vi "RailPress_PID.vi"(0 "Control Enable":bool, 1 "Fault Input":bool, 2 "Rail Press Setpoint":sgl format="%.2f", 3 "Rail Pressure":sgl format="%.2f", 5 "PID Enable":bool, 9 "PID Settings":T5={"PID_Kp"=0.0, "PID_Ti"=0.01, "PID_Td"=0.0, "PID_FF"=0.0, "Non-PID_FF"=0.0, "PID_Min"=-100.0, "PID_Max"=100.0} {"PID_Max" format="%.2f"; "PID_Min" format="%.2f"; "PID_Td" format="%.3f"; "PID_Ti" format="%.3f"}, 11 "Output Management Controls":T3, 12 "dt (s)":sgl=-1.0 format="%.3f") -> (4 "Output":T4, 14 "PID_Action_Output":T2, 15 "LS Output":T1)   [LabVIEW 2015, in "ECS-RT.lvlib"]
uses:
  ECS-RT.lvlib
  Typedefs/Raw Outputs/LS.ctl
  ECS-Shared.lvlib
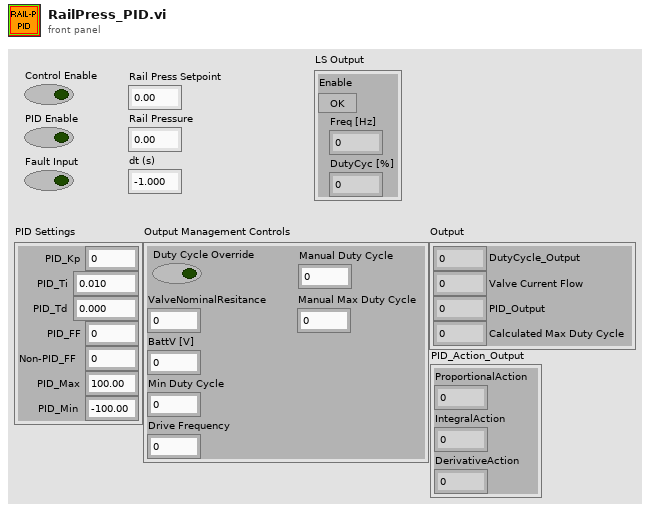
[diagram p1: front panel]
types:
  T1 = typedef "ECS-Shared.lvlib/LS.ctl" = cluster{"Enable":bool, "Freq [Hz]":sgl, "DutyCyc [%]":sgl}
  T2 = cluster{"ProportionalAction":sgl, "IntegralAction":sgl, "DerivativeAction":sgl}
  T3 = cluster{"BattV [V]":sgl, "ValveNominalResitance":sgl, "Min Duty Cycle":sgl, "Manual Max Duty Cycle":sgl, "Manual Duty Cycle":sgl, "Duty Cycle Override":bool, "Drive Frequency":sgl}
  T4 = cluster{"DutyCycle_Output":sgl, "Calculated Max Duty Cycle":sgl, "Valve Current Flow":sgl, "PID_Output":sgl}
  T5 = cluster{"PID_Kp":sgl, "PID_Ti":sgl, "PID_Td":sgl, "PID_FF":sgl, "Non-PID_FF":sgl, "PID_Min":sgl, "PID_Max":sgl}
  T6 = cluster{"DutyCycle_Output":sgl, "Max Duty Cycle":sgl, "Valve Current Flow":sgl, "PID_Output":sgl}
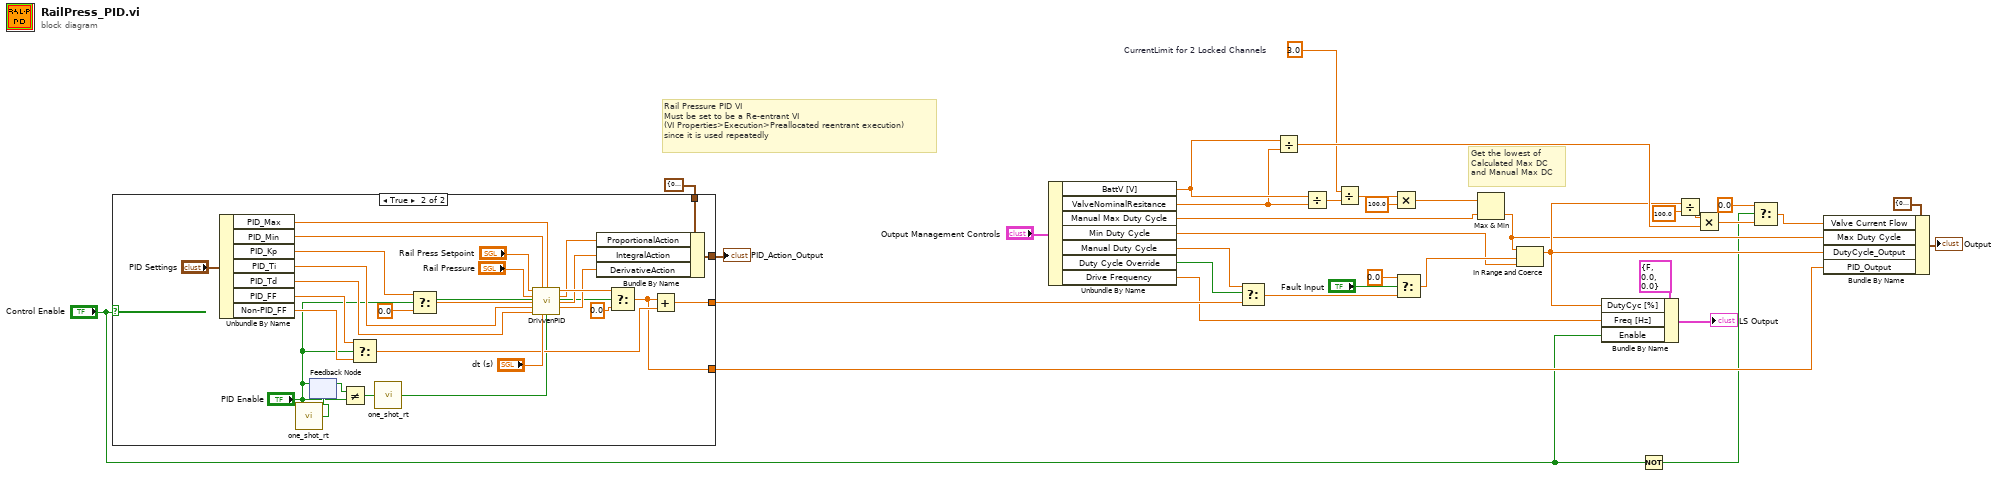
[diagram p0: block diagram]
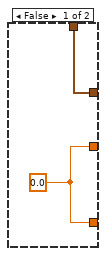
[diagram p2: hidden frame]
diagram:
  w4 = sgl 3.0  # CurrentLimit for 2 Locked Channels
  # "Rail Pressure PID VI\nMust be set to be a Re-entrant VI \n(VI Properties>Execution>Preallocated reentrant execution)\nsince it is used repeatedly"
  # "Get the lowest of \nCalculated Max DC\nand Manual Max DC"
  n1 = case shown="True" "Control Enable" {
    tunnel: [w37 w57] -> w19
    tunnel: [w37 w54] -> w23
    tunnel: T2 {"ProportionalAction"=0.0, "IntegralAction"=0.0, "DerivativeAction"=0.0} -> [w36 w43]
    tunnel: [w36 w42] -> w11
    frame False {
      w37 = sgl 0.0 ("f")
    }
    frame True {
      n2 = Unbundle By Name("PID Settings") -> ("PID_Max"=w50:sgl, "PID_Min"=w49:sgl, "PID_Kp"=w51:sgl, "PID_Ti"=w48:sgl, "PID_Td"=w47:sgl, "PID_FF"=w46:sgl, "Non-PID_FF"=w45:sgl)
      n3 = call <vilib>:"one_shot_rt.vi"("I"="PID Enable") -> ("O"=w39:bool)
      n4 = feedback #1(w39) -> (w56:bool)
      n5 = feedback-in #1("PID Enable") -> ()
      n6 = Not Equal?(x=w56, y="PID Enable") -> (x != y?=w55:bool)
      n7 = Select(t=w46, s="PID Enable", f=w45) -> (s? t:f=w60:sgl)
      n8 = call <vilib>:"one_shot_rt.vi"("I"=w55) -> ("O"=w53:bool)
      n9 = Select(t=w51, s="PID Enable", f=sgl 0.0 ("t")) -> (s? t:f=w64:sgl)
      n10 = call <vilib>:"DrivvenPID.vi"("Setpoint"="Rail Press Setpoint", "OutputLow"=w49, "OutputHigh"=w50, "ProcessVariable"="Rail Pressure", "ProportionalGain (Kc)"=w64, "IntegralTime (Ti, min)"=w48, "DerivativeTime (Td, min)"=w47, "dt (s)"="dt (s)", "Reinitialize? (F)"=w53) -> ("Output"=w59:sgl, "ProportionalAction"=w44:sgl, "IntegralAction"=w41:sgl, "DerivativeAction"=w40:sgl)  [unwired: 1 in, 2 out]
      n11 = Bundle By Name(cluster=w43, "ProportionalAction"=w44, "IntegralAction"=w41, "DerivativeAction"=w40) -> (w42:T2)
      n12 = Select(t=w59, s="PID Enable", f=sgl 0.0) -> (s? t:f=w57:sgl)
      n13 = Add(x=w57, y=w60) -> (x+y=w54:sgl)
    }
  }
  "PID_Action_Output" <- w11
  n14 = Unbundle By Name("Output Management Controls") -> ("BattV [V]"=w9:sgl, "ValveNominalResitance"=w8:sgl, "Manual Max Duty Cycle"=w6:sgl, "Min Duty Cycle"=w17:sgl, "Manual Duty Cycle"=w16:sgl, "Duty Cycle Override"=w15:bool, "Drive Frequency"=w13:sgl)
  n15 = Select(t=w16, s=w15, f=w23) -> (s? t:f=w25:sgl)
  n16 = Divide(x=w9, y=w8) -> (x/y=w32:sgl)
  n17 = Divide(x=w9, y=w8) -> (x/y=w31:sgl)
  n18 = Divide(x=w4, y=w31) -> (x/y=w30:sgl)
  n19 = Multiply(x=w30, y=sgl 100.0) -> (x*y=w7:sgl)
  n20 = Select(t=sgl 0.0, s="Fault Input", f=w25) -> (s? t:f=w24:sgl)
  n21 = Max & Min(x=w7, y=w6) -> (min(x,y)=w5:sgl)  [unwired: 1 out]
  n22 = In Range and Coerce(upper limit=w5, x=w24, lower limit=w17) -> (coerced(x)=w14:sgl)  [unwired: 1 out]
  n23 = Bundle By Name(cluster=T1 {"Enable"=FALSE, "Freq [Hz]"=0.0, "DutyCyc [%]"=0.0} ("LS Output"), "DutyCyc [%]"=w14, "Freq [Hz]"=w13, "Enable"="Control Enable") -> (→"LS Output":T1)
  n24 = Not(x="Control Enable") -> (.not. x?=w1:bool)
  n25 = Divide(x=w14, y=sgl 100.0) -> (x/y=w33:sgl)
  n26 = Multiply(x=w33, y=w32) -> (x*y=w35:sgl)
  n27 = Select(t=sgl 0.0, s=w1, f=w35) -> (s? t:f=w20:sgl)
  n28 = Bundle By Name(cluster=T6 {"DutyCycle_Output"=0.0, "Max Duty Cycle"=0.0, "Valve Current Flow"=0.0, "PID_Output"=0.0} ("Output"), "Valve Current Flow"=w20, "Max Duty Cycle"=w5, "DutyCycle_Output"=w14, "PID_Output"=w19) -> (→"Output":T6)
